vi "AutoTilt.vi"(8 "stop":bool, 9 "Begin":bool, 10 "RobotDriveDevRef":T1={"DevStatus"={"status"=FALSE, "code"=0, "source"=""}, "Motors[]"=[], "Square Inputs"=FALSE, "Max Output"=1.0, "Isochronous"=FALSE}) -> ()   [LabVIEW 2011]
uses:
  <vilib>/Rock Robotics/WPI/RobotDrive/WPI_RobotDriveDevRef.ctl
  <vilib>/Rock Robotics/WPI/MotorControl/WPI_MotorControlDeviceRef.ctl
  <vilib>/Rock Robotics/SystemInterfaces/Typedef/FPGA_TypedefDigitalModule.ctl
  <vilib>/Rock Robotics/SystemInterfaces/DIO/FPGA_DIOPWMChannel.ctl
  <vilib>/Rock Robotics/WPI/PWM/WPI_PWMDeadband.ctl
  <vilib>/Rock Robotics/WPI/CAN/Jaguar/SubVIs/WPI_CANJaguar_ControlMode.ctl
  <vilib>/Rock Robotics/WPI/PWM/WPI_PWMTransform_ConPane.ctl
panel:
  in  "Invert On/Off":bool
  in  "Time Off (MS)":dbl=10.0
  in  "time on (MS)":dbl=10.0
  in  "stop 2":bool
  in  "Calibrate":bool
  in  "Speed":dbl=-0.53
  in  "Noise Threshold":dbl=1.0
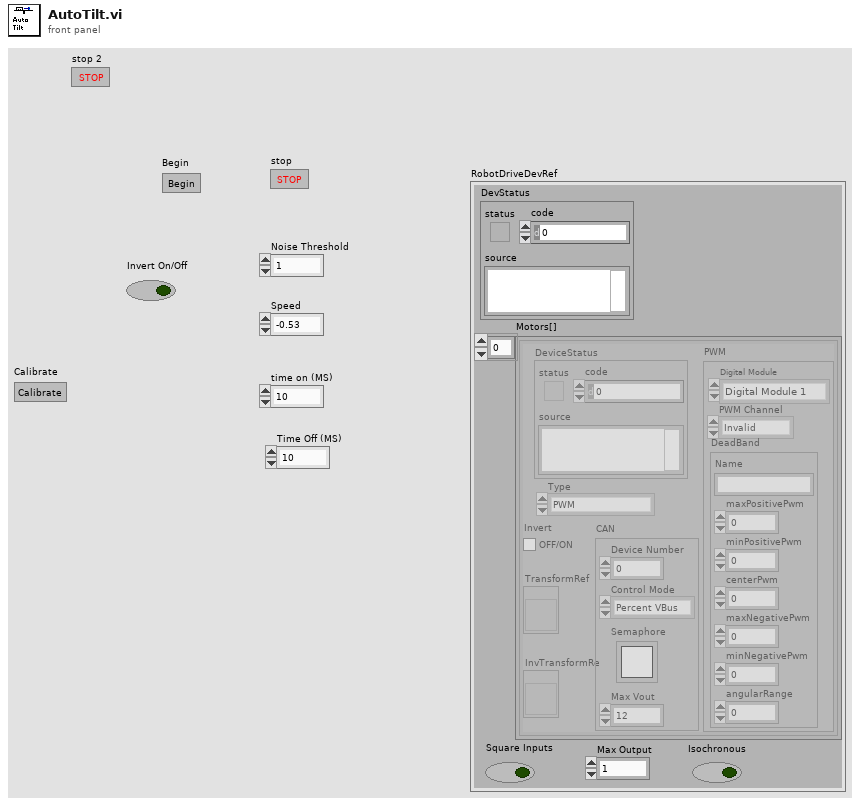
[diagram p1: front panel]
types:
  T1 = typedef "WPI_RobotDriveDevRef.ctl" = cluster{"DevStatus":errorcluster, "Motors[]":T2[], "Square Inputs":bool, "Max Output":dbl, "Isochronous":bool}
  T2 = typedef "WPI_MotorControlDeviceRef.ctl" = cluster{"DeviceStatus":errorcluster, "Type":enum16{"PWM", "CAN"}, "PWM":cluster{"Digital Module":T3, "PWM Channel":T4, "DeadBand":T5}, "CAN":cluster{"Device Number":u8, "Control Mode":T6, "Semaphore":T7, "Max Vout":dbl}, "Invert":bool, "TransformRef":T8, "InvTransformRef":T8}
  T3 = typedef "FPGA_TypedefDigitalModule.ctl" = enum16{"Digital Module 1", "Digital Module 2"}
  T4 = typedef "FPGA_DIOPWMChannel.ctl" = enum8{"PWM 1", "PWM 2", "PWM 3", "PWM 4", "PWM 5", "PWM 6", "PWM 7", "PWM 8", "PWM 9", "PWM 10", "Invalid"}
  T5 = typedef "WPI_PWMDeadband.ctl" = cluster{"Name":string, "maxPositivePwm":i32, "minPositivePwm":i32, "centerPwm":i32, "maxNegativePwm":i32, "minNegativePwm":i32, "angularRange":u16}
  T6 = typedef "WPI_CANJaguar_ControlMode.ctl" = enum8{"Percent VBus", "Current", "Speed", "Position", "Voltage"}
  T7 = typedef "Semaphore RefNum" = refnum<k1>
  T8 = typedef "WPI_PWMTransform_ConPane.ctl" = refnum<vi>
  T9 = typedef "WPI_GyroDevRef.ctl" = cluster{"DevStatus":errorcluster, "Analog Module":T10, "Analog Channel":T11, "Offset":dbl, "Gain (VoltsPerDegree/Second)":dbl}
  T10 = typedef "FPGA_TypedefAnalogModule.ctl" = enum16{"Analog Module 1", "Analog Module 2"}
  T11 = typedef "FPGA_AIChannel.ctl" = enum8{"AI 1", "AI 2", "AI 3", "AI 4", "AI 5", "AI 6", "AI 7", "AI 8", "Invalid"}
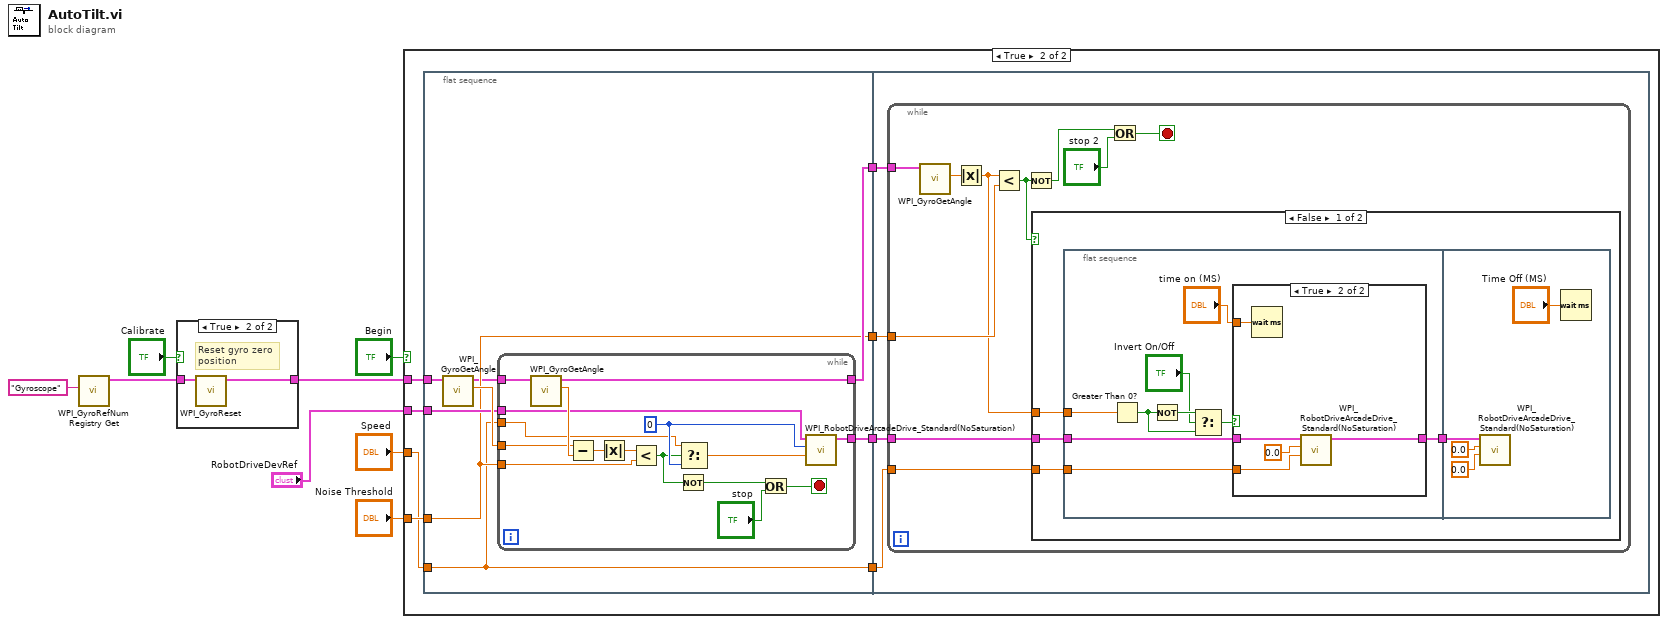
[diagram p0: block diagram]
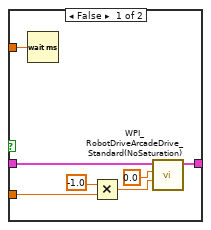
[diagram p4: hidden frame]
diagram:
  n1 = call <vilib>:"WPI_GyroRefNum Registry Get.vi"("refnum name"="Gyroscope") -> ("GyroDevRef"=w7:T9)  [unwired: 9 in, 1 out]
  n2 = case shown="True" "Calibrate" {
    tunnel: w7 -> [w9 w11]
    tunnel: [w9 w10] -> w3
    frame False {
    }
    frame True {
      # "Reset gyro zero \nposition"
      n3 = call <vilib>:"WPI_GyroReset.vi"("GyroDevRef"=w11) -> ("GyroDevRef"=w10:T9)  [unwired: 10 out]
    }
  }
  n4 = case shown="True" "Begin" {
    tunnel: w3 -> [_ w18]
    tunnel: "RobotDriveDevRef" -> [_ w19]
    tunnel: "Noise Threshold" -> [_ w17]
    tunnel: "Speed" -> [_ w14]
    frame False {
    }
    frame True {
      n5 = flat-sequence {
        tunnel: w19 -> [w26]
        tunnel: w18 -> [w25]
        tunnel: w17 -> [w23]
        tunnel: [w24] -> w16
        tunnel: [w23] -> w15
        tunnel: w14 -> [w20]
        tunnel: [w21] -> w13
        tunnel: [w20] -> w12
        tunnel: w16 -> [w47]
        tunnel: w15 -> [w46]
        tunnel: w13 -> [w45]
        tunnel: w12 -> [w44]
        frame #0 {
          n6 = call <vilib>:"WPI_GyroGetAngle.vi"("GyroDevRef"=w25) -> ("Angle"=w27:dbl, "GyroDevRef"=w22:T9)  [unwired: 1 in, 8 out]
          n7 = while {
            tunnel: w27 -> [w34]
            tunnel: w26 -> [w33]
            tunnel: w22 -> [w32]
            tunnel: w23 -> [w31]
            tunnel: [w30] -> w24
            tunnel: w20 -> [w29]
            tunnel: [w28] -> w21
            stop <- w37 stop-if-true
            w39 = 0
            n8 = call <vilib>:"WPI_GyroGetAngle.vi"("GyroDevRef"=w32) -> ("Angle"=w43:dbl, "GyroDevRef"=w30:T9)  [unwired: 1 in, 8 out]
            n9 = Subtract(x=w34, y=w43) -> (x-y=w42:dbl)
            n10 = Absolute Value(x=w42) -> (abs(x)=w41:dbl)
            n11 = Less?(x=w41, y=w31) -> (x < y?=w38:bool)
            n12 = Not(x=w38) -> (.not. x?=w36:bool)
            n13 = Select(t=w29, s=w38, f=w39) -> (s? t:f=w40:dbl)
            n14 = Or(x=w36, y="stop") -> (x .or. y?=w37:bool)
            n15 = call <vilib>:"WPI_RobotDriveArcadeDrive_Standard(NoSaturation).vi"("Y axis value"=w40, "X axis value"=w39, "RobotDriveDevRef"=w33) -> ("RobotDriveDevRef"=w28:T1)  [unwired: 1 in, 7 out]
          }
        }
        frame #1 {
          n16 = while {
            tunnel: w47 -> [w57]
            tunnel: w46 -> [w55]
            tunnel: w45 -> [w49]
            tunnel: w44 -> [w48]
            stop <- w52 stop-if-true
            n17 = call <vilib>:"WPI_GyroGetAngle.vi"("GyroDevRef"=w57) -> ("Angle"=w56:dbl)  [unwired: 1 in, 9 out]
            n18 = Absolute Value(x=w56) -> (abs(x)=w50:dbl)
            n19 = Less?(x=w50, y=w55) -> (x < y?=w51:bool)
            n20 = Not(x=w51) -> (.not. x?=w54:bool)
            n21 = case shown="False" w51 {
              tunnel: w50 -> [w61 _]
              tunnel: w49 -> [w60 _]
              tunnel: w48 -> [w59 _]
              frame False {
                n22 = flat-sequence {
                  tunnel: w61 -> [w70]
                  tunnel: w60 -> [w68]
                  tunnel: w59 -> [w67]
                  tunnel: [w66] -> w58
                  tunnel: w58 -> [w85]
                  frame #0 {
                    n23 = Greater Than 0?(x=w70) -> (x > 0?=w64:bool)
                    n24 = Not(x=w64) -> (.not. x?=w63:bool)
                    n25 = Select(t=w63, s="Invert On/Off", f=w64) -> (s? t:f=w65:bool)
                    n26 = case shown="True" w65 {
                      tunnel: "time on (MS)" -> [w76 w82]
                      tunnel: w68 -> [w75 w81]
                      tunnel: w67 -> [w73 w79]
                      tunnel: [w71 w78] -> w66
                      frame False {
                        n27 = Wait (ms)(milliseconds to wait=w76) -> ()  [unwired: 1 out]
                        n28 = Multiply(x=-1.0, y=w73) -> (x*y=w72:dbl)
                        n29 = call <vilib>:"WPI_RobotDriveArcadeDrive_Standard(NoSaturation).vi"("Y axis value"=w72, "X axis value"=0.0, "RobotDriveDevRef"=w75) -> ("RobotDriveDevRef"=w71:T1)  [unwired: 1 in, 7 out]
                      }
                      frame True {
                        n30 = Wait (ms)(milliseconds to wait=w82) -> ()  [unwired: 1 out]
                        n31 = call <vilib>:"WPI_RobotDriveArcadeDrive_Standard(NoSaturation).vi"("Y axis value"=w79, "X axis value"=0.0, "RobotDriveDevRef"=w81) -> ("RobotDriveDevRef"=w78:T1)  [unwired: 1 in, 7 out]
                      }
                    }
                  }
                  frame #1 {
                    n32 = call <vilib>:"WPI_RobotDriveArcadeDrive_Standard(NoSaturation).vi"("Y axis value"=0.0, "X axis value"=0.0, "RobotDriveDevRef"=w85) -> ()  [unwired: 1 in, 8 out]
                    n33 = Wait (ms)(milliseconds to wait="Time Off (MS)") -> ()  [unwired: 1 out]
                  }
                }
              }
              frame True {
              }
            }
            n34 = Or(x=w54, y="stop 2") -> (x .or. y?=w52:bool)
          }
        }
      }
    }
  }
